vi "SetExposure.vi"(8 "error in (no error)":errorcluster, 10 "Arg":string, 11 "ThorLabsCsCamera in":refnum<class "ThorLabsCsCamera.lvclass">) -> (0 "error out":errorcluster, 2 "setValue out":dbl, 3 "ThorLabsCsCamera out":refnum<class "ThorLabsCsCamera.lvclass">)   [LabVIEW 2020, in "ThorLabsCsCamera.lvclass"]
uses:
  ThorLabsCsCamera.lvclass
  ThorLabsCsCamera.lvclass/ThorLabsCsCamera.ctl
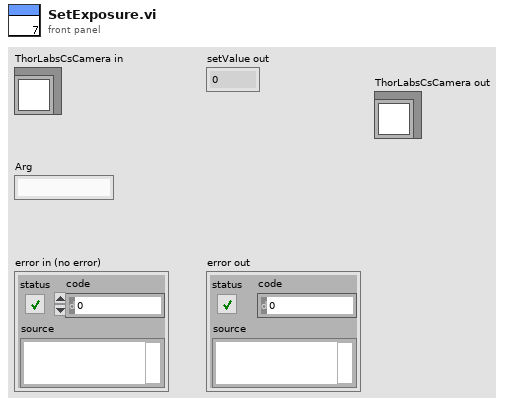
[diagram p1: front panel]
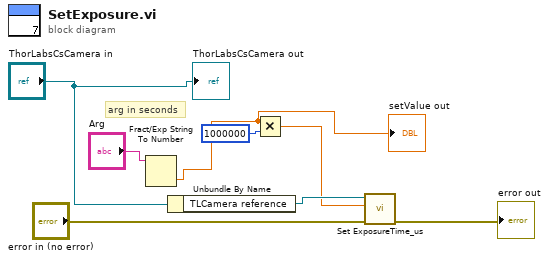
[diagram p0: block diagram]
diagram:
  # "arg in seconds"
  n1 = Fract/Exp String To Number(string="Arg") -> (number=w1:dbl)  [unwired: 3 in, 1 out]
  "setValue out" <- w1
  n2 = Unbundle By Name("ThorLabsCsCamera in") -> ("TLCamera reference"=w4:refnum<k24>)
  n3 = Multiply(x=w1, y=u32 1000000) -> (x*y=w3:dbl)
  n4 = call "Set ExposureTime_us.vi"("error in (no error)"="error in (no error)", "ExposureTime_us"=w3, "TLCamera reference in"=w4) -> ("error out"=→"error out":errorcluster)  [unwired: 7 in, 1 out]
  "ThorLabsCsCamera out" <- "ThorLabsCsCamera in"
